vi "NI VeriStand - Get Aliases.vi"(8 "Error in":errorcluster, 11 "Runtime Configuration Ref in":refnum<k39>) -> (0 "Error out":errorcluster, 1 "Alias Names":string[](array[string]), 2 "Referenced Channels":string[](array[string]), 3 "Runtime Configuration Ref out":refnum<k39>, 4 "Success":bool, 5 "Runtime Alias Folder Name":string)   [LabVIEW 2025, in "Runtime Configuration File API.lvlib"]
uses:
  Runtime Configuration File API.lvlib
  C:/NetCoreDLL/NationalInstruments.VeriStand.SystemDefinitionAPI.dll
  NetCoreDLL/NationalInstruments.VeriStand.SystemDefinitionAPI.dll
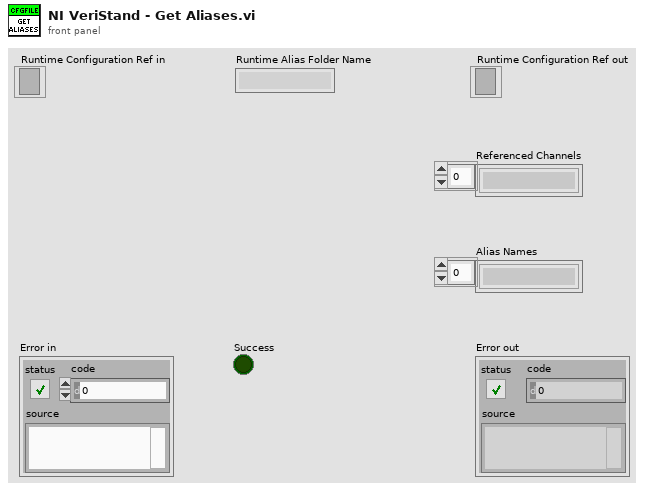
[diagram p1: front panel]
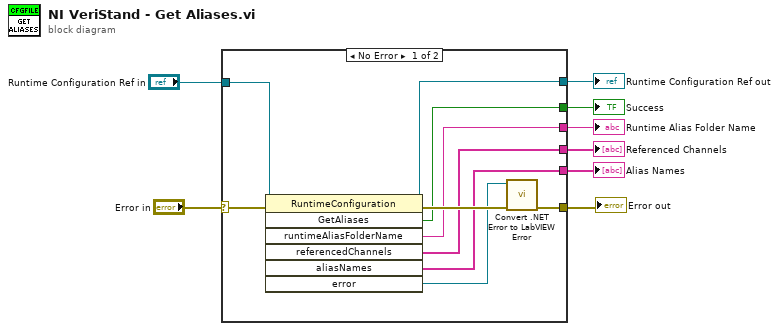
[diagram p0: block diagram]
diagram:
  n1 = case shown="No Error" "Error in" {
    selector: "Error in" -> [w18 w19]
    tunnel: "Runtime Configuration Ref in" -> [w15 _]
    tunnel: [w14 _] -> w5
    tunnel: [w16 w19] -> w8
    tunnel: [w13 _] -> w4
    tunnel: [w12 _] -> w3
    tunnel: [w11 _] -> w2
    tunnel: [w10 _] -> w1
    frame No Error {
      n2 = invoke class="RuntimeConfiguration" method="GetAliases"(reference=w15, error in=w18) -> (reference out=w14:refnum<k39>, error out=w17:errorcluster, "GetAliases"=w13:bool, "runtimeAliasFolderName"=w12:string, "referencedChannels"=w11:string[], "aliasNames"=w10:string[], "error"=w9:refnum<k39>)  [unwired: 5 in]
      n3 = call "Convert .NET Error to LabVIEW Error.vi"("error in"=w17, "NationalInstruments.VeriStand.Error"=w9) -> ("error out"=w16:errorcluster)  [unwired: 9 in]
    }
    frame Error {
    }
  }
  "Runtime Configuration Ref out" <- w5
  "Error out" <- w8
  "Success" <- w4
  "Referenced Channels" <- w2
  "Alias Names" <- w1
  "Runtime Alias Folder Name" <- w3
